vi "Sub_Wait.vi"(8 "error in (no error)":errorcluster, 10 "milliseconds to wait":u32=1000, 11 "connection ID":refnum<k5>) -> (0 "error out":errorcluster, 3 "connection ID out":refnum<k5>)   [LabVIEW 2020, in "MQTT_Functions.lvlib"]
uses:
  MQTT_Functions.lvlib
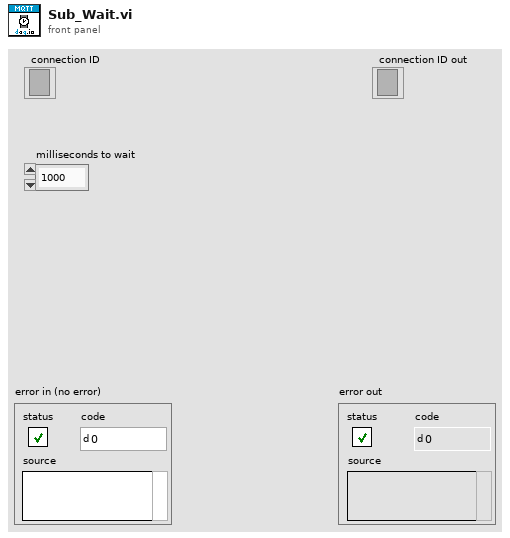
[diagram p1: front panel]
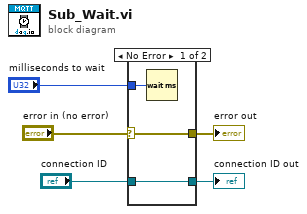
[diagram p0: block diagram]
diagram:
  n1 = case shown="No Error" "error in (no error)" {
    selector: "error in (no error)" -> [w8 w10]
    tunnel: [w8 w10] -> w4
    tunnel: "connection ID" -> [w7 w9]
    tunnel: [w7 w9] -> w2
    tunnel: "milliseconds to wait" -> [w6 _]
    frame No Error {
      n2 = Wait (ms)(milliseconds to wait=w6) -> ()  [unwired: 1 out]
    }
    frame Error {
    }
  }
  "connection ID out" <- w2
  "error out" <- w4
